vi "Ubidots_GET.vi"() -> ()   [LabVIEW 2016]
doc: "Use this template to simulate the generation and display of data.\nNote: LabVIEW enables automatic error handling by default for VIs you create from this template."
uses:
  <vilib>/httpClient/LabVIEWHTTPClient.lvlib
panel:
  out "Gauge":dbl(knob) scale=-10.0..10.0 scale format="%#_2g"
  out "Value:":string
  in  "stop":bool
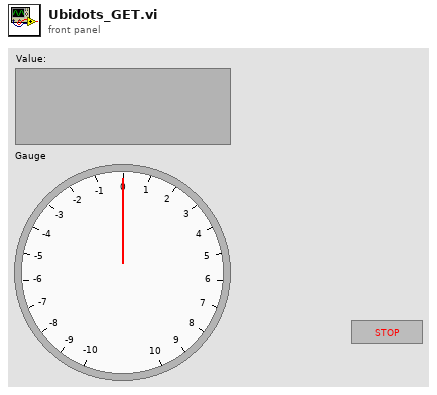
[diagram p1: front panel]
types:
  T1 = typedef "LabVIEWHTTPClient.lvlib/ClientHandle.ctl" = refnum<k1>
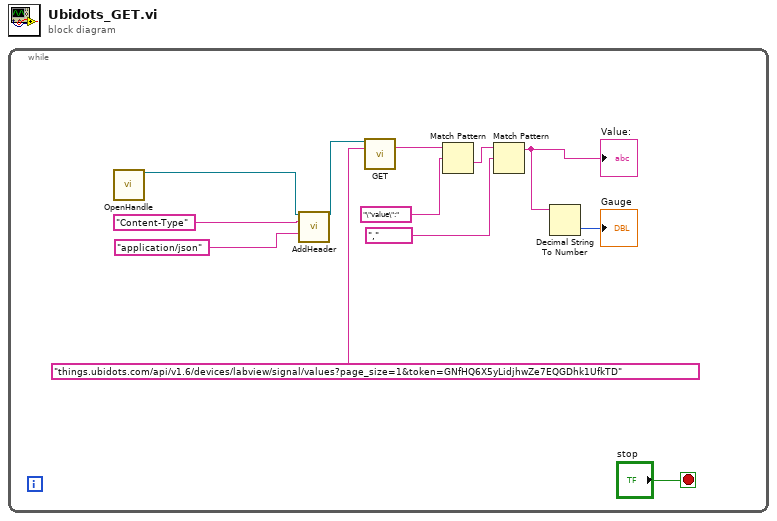
[diagram p0: block diagram]
diagram:
  n1 = while {
    stop <- "stop" stop-if-true
    n2 = call <vilib>:"OpenHandle.vi"() -> ("client handle out"=w9:T1)  [unwired: 14 in, 1 out]
    n3 = call <vilib>:"AddHeader.vi"("client handle"=w9, "header"="Content-Type", "value"="application/json") -> ("client handle out"=w8:T1)  [unwired: 11 in, 1 out]
    n4 = call <vilib>:"GET.vi"("client handle"=w8, "url"="things.ubidots.com/api/v1.6/devices/labview/signal/values?page_size=1&token=GNfHQ6X5yLidjhwZe7EQGDhk1UfkTD") -> ("body"=w3:string)  [unwired: 10 in, 3 out]
    n5 = Match Pattern(string=w3, regular expression="\"value\":") -> (after substring=w5:string)  [unwired: 1 in, 3 out]
    n6 = Match Pattern(string=w5, regular expression=",") -> (before substring=w1:string)  [unwired: 1 in, 3 out]
    "Value:" <- w1
    n7 = Decimal String To Number(string=w1) -> (number=→"Gauge":i32)  [unwired: 2 in, 1 out]
  }
